vi "Namen fuer File erzeugen.vi"(11 "String Eingabe":T1) -> (1 "File Name LIN":string, 3 "File Name EPA":string)   [LabVIEW 2020, in "Linearisierung v2.lvlib"]
uses:
  Linearisierung v2.lvlib
  Visualisierungs Elemente/String - Eingabefeld.ctl
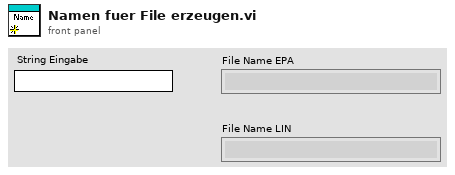
[diagram p1: front panel]
types:
  T1 = typedef "String - Eingabefeld.ctl" = string
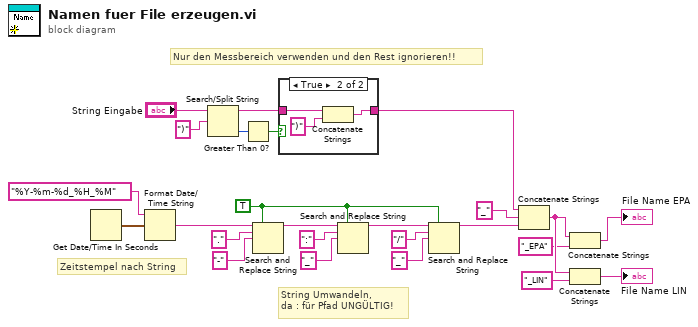
[diagram p0: block diagram]
diagram:
  w14 = TRUE ("Alle ersetzen? (F)")
  # "Nur den Messbereich verwenden und den Rest ignorieren!!"
  # "String Umwandeln, \nda : für Pfad UNGÜLTIG!"
  # "Zeitstempel nach String"
  n1 = Get Date/Time In Seconds() -> (seconds since 1Jan1904=w25:timestamp)
  n2 = Format Date/Time String(time format string (%c)="%Y-%m-%d_%H_%M" ("Zeitformatierungs-String (%c)"), seconds (now)=w25) -> (date/time string=w24:string)  [unwired: 1 in]
  n3 = Search/Split String(string="String Eingabe", search string/char (-)=")" ("Nach String/Zeichen suchen (-)")) -> (substring before match=w7:T1, offset of match=w9:i32)  [unwired: 1 in, 1 out]
  n4 = Greater Than 0?(x=w9) -> (x > 0?=w8:bool)
  n5 = Search and Replace String(replace all?=w14, input string=w24, search string="." ("Such-String"), replace string="-" ("String ersetzen(\"\")")) -> (result string=w21:string)  [unwired: 4 in, 3 out]
  n6 = case shown="True" w8 {
    tunnel: w7 -> [w26 w29]
    tunnel: [w26 w28] -> w6
    frame False {
    }
    frame True {
      n7 = Concatenate Strings(w29, ")" ("String")) -> (w28:string)
    }
  }
  n8 = Search and Replace String(replace all?=w14, input string=w21, search string=":" ("Such-String"), replace string="_" ("String ersetzen(\"\")")) -> (result string=w15:string)  [unwired: 4 in, 3 out]
  n9 = Search and Replace String(replace all?=w14, input string=w15, search string="/" ("Such-String"), replace string="_" ("String ersetzen(\"\")")) -> (result string=w13:string)  [unwired: 4 in, 3 out]
  n10 = Concatenate Strings(w6, "_", w13) -> (w3:string)
  n11 = Concatenate Strings(w3, "_EPA" ("String")) -> (→"File Name EPA":string)
  n12 = Concatenate Strings(w3, "_LIN" ("String")) -> (→"File Name LIN":string)
